vi "De_RateMatch_Turbo.vi"(4 "error in (no error)":errorcluster caption="错误输入（无错误）", 6 "EN_LDPC":dbl, 7 "Zc":dbl, 8 "dermdata":dbl[][](array[numeric]), 9 "H":dbl, 10 "C":dbl, 11 "appended path":path) -> (0 "error IO":errorcluster, 5 "deldpccode":dbl[][](array[numeric]))   [LabVIEW 2015]
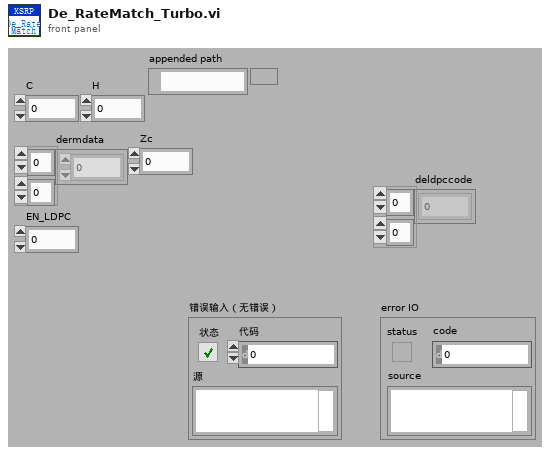
[diagram p1: front panel]
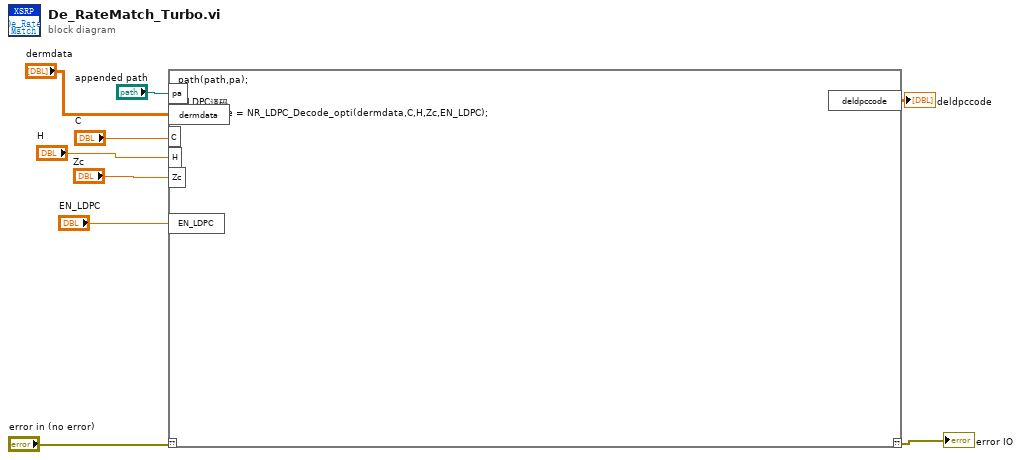
[diagram p0: block diagram]
diagram:
  n1 = script code="path(path,pa);\n\n%LDPC译码\ndeldpccode = NR_LDPC_Decode_opti(dermdata,C,H,Zc,EN_LDPC);"("??"="error in (no error)", "pa"="appended path", "dermdata"="dermdata", "C"="C", "H"="H", "Zc"="Zc", "EN_LDPC"="EN_LDPC") -> ("??"=→"error IO":errorcluster, "deldpccode"=→"deldpccode":dbl[][])
